vi "Wyciągnięcie z tekstu współrzędnej punktu w formacie dziesiętnym.vi"(7 "Format wprowadzanej współrzędnej":i8, 8 "Współrzędna w postaci tekstowej":string) -> (0 "error constant":errorcluster, 3 "Szerokość geograficzna (NS)":dbl format="%#.6g", 5 "Długość geograficzna (EW)":dbl format="%#.6g")   [LabVIEW 2015, in "Biblioteka moduł map v3.lvlib" / "Konwersja wsp.lvlib"]
doc: "Przed użyciem subVI należy \"wyznaczyć format wprowadzanej współrzędnej\". Dopiero później można użyć subVI, gdyż algorytm zakłada prawidłowe wprowadzenie współrzędnych.\n\nWprowadzana jest współrzędna w postaci tekstowej oraz format wprowadzanej współrzędnej (D, DM, DMS). W zależności od formatu dokonywana jest konwersja współrzędnej w postaci tekstowej na dwie współrzedne podające wartość długoścci i szerokości geograficznej jako wartości dziesiętne. s"
uses:
  Konwersja wsp.lvlib
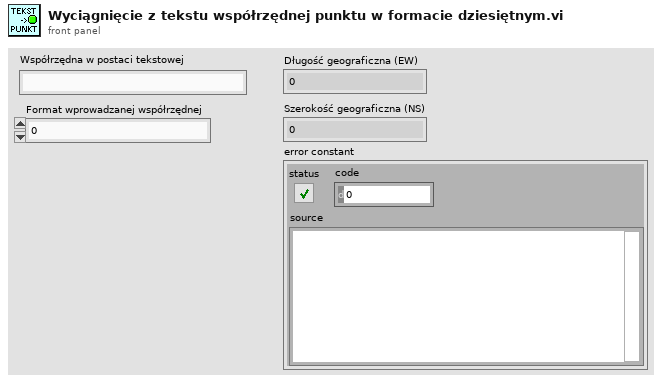
[diagram p1: front panel]
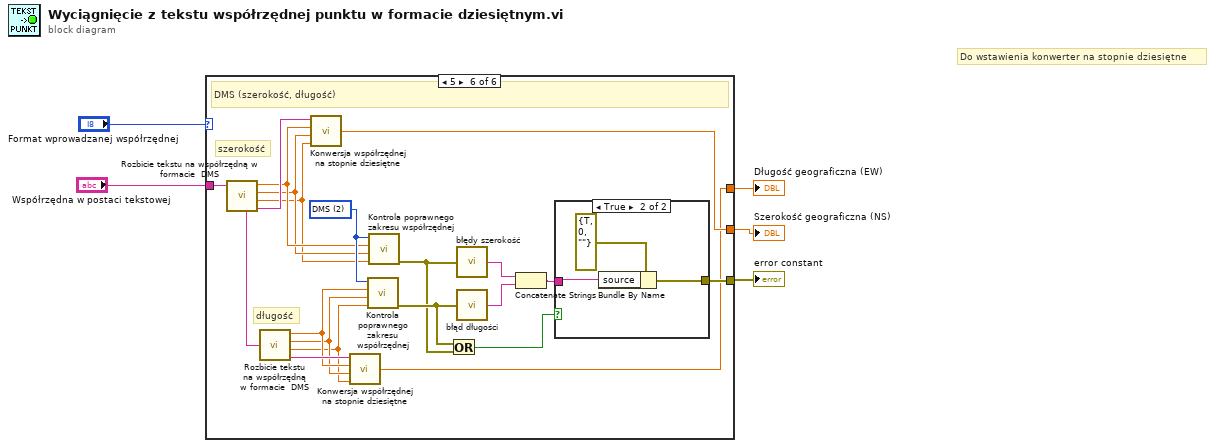
[diagram p0: block diagram]
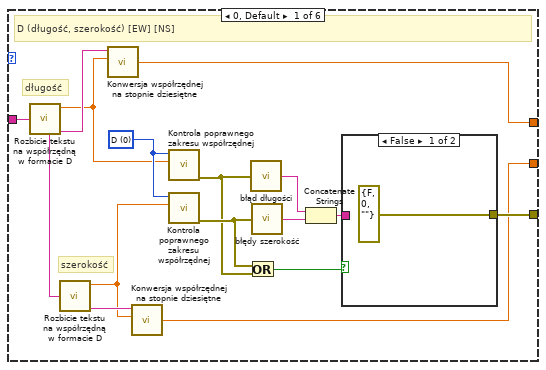
[diagram p2: hidden frame]
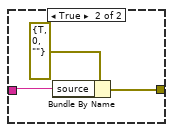
[diagram p3: hidden frame]
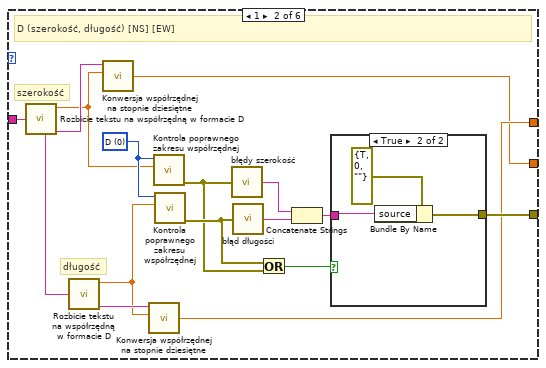
[diagram p4: hidden frame]
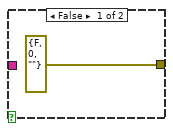
[diagram p5: hidden frame]
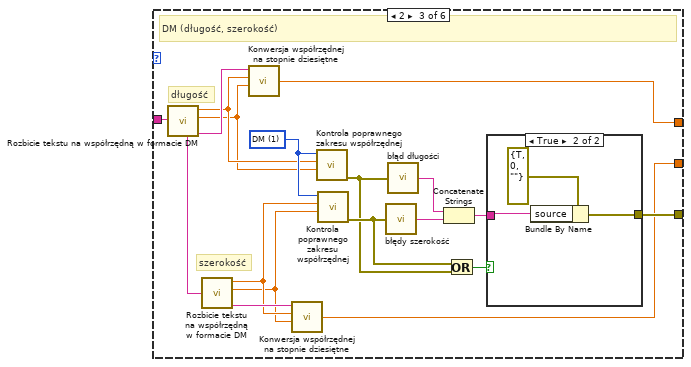
[diagram p6: hidden frame]
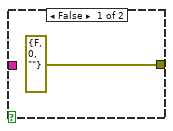
[diagram p7: hidden frame]
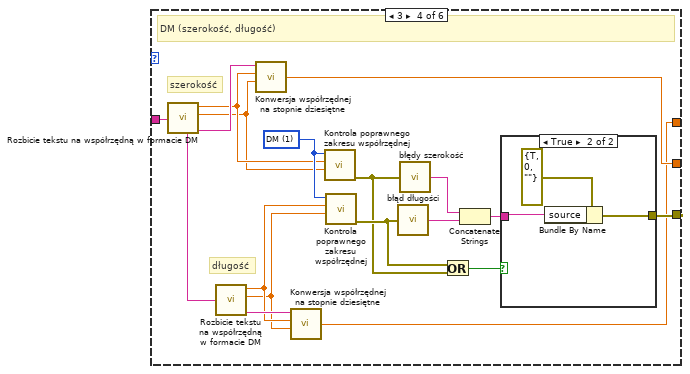
[diagram p8: hidden frame]
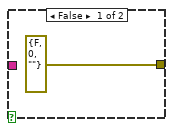
[diagram p9: hidden frame]
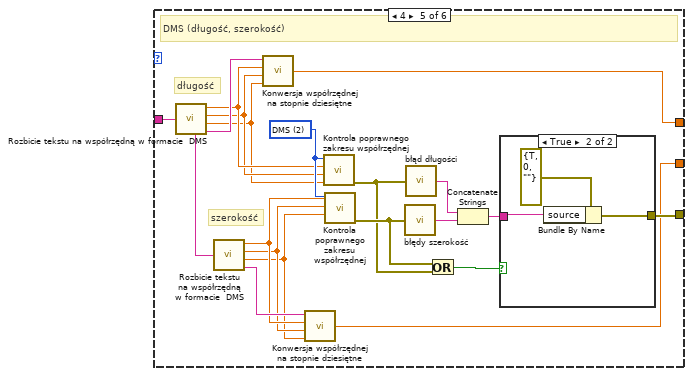
[diagram p10: hidden frame]
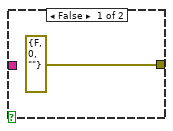
[diagram p11: hidden frame]
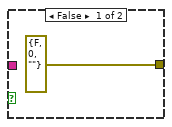
[diagram p12: hidden frame]
diagram:
  # "Do wstawienia konwerter na stopnie dziesiętne"
  n1 = case shown="5" "Format wprowadzanej współrzędnej" {
    tunnel: "Współrzędna w postaci tekstowej" -> [w16 w41 w63 w85 w109 w133]
    tunnel: [w17 w32 w54 w76 w101 w125] -> w1
    tunnel: [w6 w27 w50 w68 w91 w115] -> w3
    tunnel: [w7 w26 w47 w69 w90 w116] -> w2
    frame 0, Default {
      w21 = u16 0 items=["D", "DM", "DMS"] ("Format współrzędnych")
      # "długość"
      # "szerokość"
      # "D (długość, szerokość) [EW] [NS]"
      n2 = call "Rozbicie tekstu na współrzędną w formacie D.vi"("Współrzędna tekstowa"=w16) -> ("Druga współrzędna"=w15:string, "D"=w9:dbl, "Kierunek"=w11:string)  [unwired: 3 in]
      n3 = call "Rozbicie tekstu na współrzędną w formacie D.vi"("Współrzędna tekstowa"=w15) -> ("D"=w8:dbl, "Kierunek"=w10:string)  [unwired: 3 in, 1 out]
      n4 = call "Konwersja współrzędnej na stopnie dziesiętne.vi"("Kierunek"=w11, "D"=w9) -> ("Współrzędna dziesiętna"=w6:ext)  [unwired: 6 in]
      n5 = call "Konwersja współrzędnej na stopnie dziesiętne.vi"("Kierunek"=w10, "D"=w8) -> ("Współrzędna dziesiętna"=w7:ext)  [unwired: 6 in]
      n6 = call "Kontrola poprawnego zakresu współrzędnej.vi"("Stopnie"=w9, "Format współrzędnych"=w21) -> ("error constant"=w18:errorcluster)  [unwired: 9 in]
      n7 = call "Kontrola poprawnego zakresu współrzędnej.vi"("Stopnie"=w8, "Format współrzędnych"=w21) -> ("error constant"=w19:errorcluster)  [unwired: 9 in]
      n8 = Or(x=w19, y=w18) -> (x .or. y?=w13:bool)
      n9 = call "błąd długości.vi"("błąd długości"=w18) -> ("Błędy długości"=w20:string)  [unwired: 4 in]
      n10 = call "błędy szerokość.vi"("błąd szerokość"=w19) -> ("Błędy  szerokości"=w12:string)  [unwired: 4 in]
      n11 = Concatenate Strings(w20, w12) -> (w14:string)
      n12 = case shown="False" w13 {
        tunnel: [errorcluster {"status"=FALSE, "code"=0, "source"=""} ("error constant") w24] -> w17
        tunnel: w14 -> [_ w23]
        frame False {
        }
        frame True {
          n13 = Bundle By Name(cluster=errorcluster {"status"=TRUE, "code"=0, "source"=""} ("error constant"), "source"=w23) -> (w24:errorcluster)
        }
      }
    }
    frame 1 {
      w39 = u16 0 items=["D", "DM", "DMS"] ("Format współrzędnych")
      # "długość"
      # "szerokość"
      # "D (szerokość, długość) [NS] [EW]"
      n14 = call "Rozbicie tekstu na współrzędną w formacie D.vi"("Współrzędna tekstowa"=w41) -> ("Druga współrzędna"=w40:string, "D"=w29:dbl, "Kierunek"=w31:string)  [unwired: 3 in]
      n15 = call "Rozbicie tekstu na współrzędną w formacie D.vi"("Współrzędna tekstowa"=w40) -> ("D"=w28:dbl, "Kierunek"=w30:string)  [unwired: 3 in, 1 out]
      n16 = call "Konwersja współrzędnej na stopnie dziesiętne.vi"("Kierunek"=w31, "D"=w29) -> ("Współrzędna dziesiętna"=w26:ext)  [unwired: 6 in]
      n17 = call "Konwersja współrzędnej na stopnie dziesiętne.vi"("Kierunek"=w30, "D"=w28) -> ("Współrzędna dziesiętna"=w27:ext)  [unwired: 6 in]
      n18 = call "Kontrola poprawnego zakresu współrzędnej.vi"("Stopnie"=w29, "Format współrzędnych"=w39) -> ("error constant"=w34:errorcluster)  [unwired: 9 in]
      n19 = call "Kontrola poprawnego zakresu współrzędnej.vi"("Stopnie"=w28, "Format współrzędnych"=w39) -> ("error constant"=w36:errorcluster)  [unwired: 9 in]
      n20 = call "błędy szerokość.vi"("błąd szerokość"=w34) -> ("Błędy  szerokości"=w33:string)  [unwired: 4 in]
      n21 = call "błąd długości.vi"("błąd długości"=w36) -> ("Błędy długości"=w35:string)  [unwired: 4 in]
      n22 = Or(x=w36, y=w34) -> (x .or. y?=w37:bool)
      n23 = Concatenate Strings(w33, w35) -> (w38:string)
      n24 = case shown="True" w37 {
        tunnel: [errorcluster {"status"=FALSE, "code"=0, "source"=""} ("error constant") w44] -> w32
        tunnel: w38 -> [_ w43]
        frame False {
        }
        frame True {
          n25 = Bundle By Name(cluster=errorcluster {"status"=TRUE, "code"=0, "source"=""} ("error constant"), "source"=w43) -> (w44:errorcluster)
        }
      }
    }
    frame 2 {
      w55 = u16 1 items=["D", "DM", "DMS"] ("Format współrzędnych")
      # "szerokość"
      # "długość"
      # "DM (długość, szerokość)"
      n26 = call "Rozbicie tekstu na współrzędną w formacie DM.vi"("Współrzędna tekstowa"=w63) -> ("Kierunek"=w53:string, "Druga współrzędna"=w62:string, "M"=w51:dbl, "D"=w52:dbl)  [unwired: 4 in]
      n27 = call "Rozbicie tekstu na współrzędną w formacie DM.vi"("Współrzędna tekstowa"=w62) -> ("Kierunek"=w49:string, "M"=w46:dbl, "D"=w48:dbl)  [unwired: 4 in, 1 out]
      n28 = call "Konwersja współrzędnej na stopnie dziesiętne.vi"("Kierunek"=w53, "D"=w52, "M"=w51) -> ("Współrzędna dziesiętna"=w50:ext)  [unwired: 5 in]
      n29 = call "Konwersja współrzędnej na stopnie dziesiętne.vi"("Kierunek"=w49, "D"=w48, "M"=w46) -> ("Współrzędna dziesiętna"=w47:ext)  [unwired: 5 in]
      n30 = call "Kontrola poprawnego zakresu współrzędnej.vi"("Minuty"=w51, "Stopnie"=w52, "Format współrzędnych"=w55) -> ("error constant"=w59:errorcluster)  [unwired: 8 in]
      n31 = call "Kontrola poprawnego zakresu współrzędnej.vi"("Minuty"=w46, "Stopnie"=w48, "Format współrzędnych"=w55) -> ("error constant"=w60:errorcluster)  [unwired: 8 in]
      n32 = call "błędy szerokość.vi"("błąd szerokość"=w60) -> ("Błędy  szerokości"=w56:string)  [unwired: 4 in]
      n33 = call "błąd długości.vi"("błąd długości"=w59) -> ("Błędy długości"=w61:string)  [unwired: 4 in]
      n34 = Concatenate Strings(w61, w56) -> (w58:string)
      n35 = Or(x=w60, y=w59) -> (x .or. y?=w57:bool)
      n36 = case shown="True" w57 {
        tunnel: [errorcluster {"status"=FALSE, "code"=0, "source"=""} ("error constant") w66] -> w54
        tunnel: w58 -> [_ w65]
        frame False {
        }
        frame True {
          n37 = Bundle By Name(cluster=errorcluster {"status"=TRUE, "code"=0, "source"=""} ("error constant"), "source"=w65) -> (w66:errorcluster)
        }
      }
    }
    frame 3 {
      w77 = u16 1 items=["D", "DM", "DMS"] ("Format współrzędnych")
      # "długość"
      # "szerokość"
      # "DM (szerokość, długość)"
      n38 = call "Rozbicie tekstu na współrzędną w formacie DM.vi"("Współrzędna tekstowa"=w85) -> ("Kierunek"=w75:string, "Druga współrzędna"=w84:string, "M"=w73:dbl, "D"=w74:dbl)  [unwired: 4 in]
      n39 = call "Rozbicie tekstu na współrzędną w formacie DM.vi"("Współrzędna tekstowa"=w84) -> ("Kierunek"=w72:string, "M"=w70:dbl, "D"=w71:dbl)  [unwired: 4 in, 1 out]
      n40 = call "Konwersja współrzędnej na stopnie dziesiętne.vi"("Kierunek"=w75, "D"=w74, "M"=w73) -> ("Współrzędna dziesiętna"=w69:ext)  [unwired: 5 in]
      n41 = call "Konwersja współrzędnej na stopnie dziesiętne.vi"("Kierunek"=w72, "D"=w71, "M"=w70) -> ("Współrzędna dziesiętna"=w68:ext)  [unwired: 5 in]
      n42 = call "Kontrola poprawnego zakresu współrzędnej.vi"("Minuty"=w73, "Stopnie"=w74, "Format współrzędnych"=w77) -> ("error constant"=w79:errorcluster)  [unwired: 8 in]
      n43 = call "Kontrola poprawnego zakresu współrzędnej.vi"("Minuty"=w70, "Stopnie"=w71, "Format współrzędnych"=w77) -> ("error constant"=w81:errorcluster)  [unwired: 8 in]
      n44 = call "błąd długości.vi"("błąd długości"=w81) -> ("Błędy długości"=w80:string)  [unwired: 4 in]
      n45 = call "błędy szerokość.vi"("błąd szerokość"=w79) -> ("Błędy  szerokości"=w78:string)  [unwired: 4 in]
      n46 = Or(x=w81, y=w79) -> (x .or. y?=w82:bool)
      n47 = Concatenate Strings(w78, w80) -> (w83:string)
      n48 = case shown="True" w82 {
        tunnel: [errorcluster {"status"=FALSE, "code"=0, "source"=""} ("error constant") w88] -> w76
        tunnel: w83 -> [_ w87]
        frame False {
        }
        frame True {
          n49 = Bundle By Name(cluster=errorcluster {"status"=TRUE, "code"=0, "source"=""} ("error constant"), "source"=w87) -> (w88:errorcluster)
        }
      }
    }
    frame 4 {
      w102 = u16 2 items=["D", "DM", "DMS"] ("Format współrzędnych")
      # "szerokość"
      # "długość"
      # "DMS (długość, szerokość)"
      n50 = call "Rozbicie tekstu na współrzędną w formacie  DMS.vi"("Współrzędna tekstowa"=w109) -> ("Kierunek"=w99:string, "Druga współrzędna"=w100:string, "S"=w95:dbl, "M"=w96:dbl, "D"=w97:dbl)  [unwired: 3 in]
      n51 = call "Rozbicie tekstu na współrzędną w formacie  DMS.vi"("Współrzędna tekstowa"=w100) -> ("Kierunek"=w98:string, "S"=w92:dbl, "M"=w93:dbl, "D"=w94:dbl)  [unwired: 3 in, 1 out]
      n52 = call "Konwersja współrzędnej na stopnie dziesiętne.vi"("Kierunek"=w99, "D"=w97, "M"=w96, "S"=w95) -> ("Współrzędna dziesiętna"=w91:ext)  [unwired: 4 in]
      n53 = call "Konwersja współrzędnej na stopnie dziesiętne.vi"("Kierunek"=w98, "D"=w94, "M"=w93, "S"=w92) -> ("Współrzędna dziesiętna"=w90:ext)  [unwired: 4 in]
      n54 = call "Kontrola poprawnego zakresu współrzędnej.vi"("Sekundy"=w95, "Minuty"=w96, "Stopnie"=w97, "Format współrzędnych"=w102) -> ("error constant"=w106:errorcluster)  [unwired: 7 in]
      n55 = call "Kontrola poprawnego zakresu współrzędnej.vi"("Sekundy"=w92, "Minuty"=w93, "Stopnie"=w94, "Format współrzędnych"=w102) -> ("error constant"=w107:errorcluster)  [unwired: 7 in]
      n56 = call "błędy szerokość.vi"("błąd szerokość"=w107) -> ("Błędy  szerokości"=w103:string)  [unwired: 4 in]
      n57 = call "błąd długości.vi"("błąd długości"=w106) -> ("Błędy długości"=w108:string)  [unwired: 4 in]
      n58 = Or(x=w107, y=w106) -> (x .or. y?=w104:bool)
      n59 = Concatenate Strings(w108, w103) -> (w105:string)
      n60 = case shown="True" w104 {
        tunnel: [errorcluster {"status"=FALSE, "code"=0, "source"=""} ("error constant") w112] -> w101
        tunnel: w105 -> [_ w111]
        frame False {
        }
        frame True {
          n61 = Bundle By Name(cluster=errorcluster {"status"=TRUE, "code"=0, "source"=""} ("error constant"), "source"=w111) -> (w112:errorcluster)
        }
      }
    }
    frame 5 {
      w126 = u16 2 items=["D", "DM", "DMS"] ("Format współrzędnych")
      # "długość"
      # "szerokość"
      # "DMS (szerokość, długość)"
      n62 = call "Rozbicie tekstu na współrzędną w formacie  DMS.vi"("Współrzędna tekstowa"=w133) -> ("Kierunek"=w123:string, "Druga współrzędna"=w124:string, "S"=w114:dbl, "M"=w121:dbl, "D"=w122:dbl)  [unwired: 3 in]
      n63 = call "Rozbicie tekstu na współrzędną w formacie  DMS.vi"("Współrzędna tekstowa"=w124) -> ("Kierunek"=w120:string, "S"=w117:dbl, "M"=w118:dbl, "D"=w119:dbl)  [unwired: 3 in, 1 out]
      n64 = call "Konwersja współrzędnej na stopnie dziesiętne.vi"("Kierunek"=w123, "D"=w122, "M"=w121, "S"=w114) -> ("Współrzędna dziesiętna"=w116:ext)  [unwired: 4 in]
      n65 = call "Konwersja współrzędnej na stopnie dziesiętne.vi"("Kierunek"=w120, "D"=w119, "M"=w118, "S"=w117) -> ("Współrzędna dziesiętna"=w115:ext)  [unwired: 4 in]
      n66 = call "Kontrola poprawnego zakresu współrzędnej.vi"("Sekundy"=w117, "Minuty"=w118, "Stopnie"=w119, "Format współrzędnych"=w126) -> ("error constant"=w130:errorcluster)  [unwired: 7 in]
      n67 = call "Kontrola poprawnego zakresu współrzędnej.vi"("Sekundy"=w114, "Minuty"=w121, "Stopnie"=w122, "Format współrzędnych"=w126) -> ("error constant"=w128:errorcluster)  [unwired: 7 in]
      n68 = Or(x=w130, y=w128) -> (x .or. y?=w131:bool)
      n69 = call "błędy szerokość.vi"("błąd szerokość"=w128) -> ("Błędy  szerokości"=w127:string)  [unwired: 4 in]
      n70 = call "błąd długości.vi"("błąd długości"=w130) -> ("Błędy długości"=w129:string)  [unwired: 4 in]
      n71 = Concatenate Strings(w127, w129) -> (w132:string)
      n72 = case shown="True" w131 {
        tunnel: [errorcluster {"status"=FALSE, "code"=0, "source"=""} ("error constant") w136] -> w125
        tunnel: w132 -> [_ w135]
        frame False {
        }
        frame True {
          n73 = Bundle By Name(cluster=errorcluster {"status"=TRUE, "code"=0, "source"=""} ("error constant"), "source"=w135) -> (w136:errorcluster)
        }
      }
    }
  }
  "Długość geograficzna (EW)" <- w3
  "Szerokość geograficzna (NS)" <- w2
  "error constant" <- w1
